vi "simulacao_robo_movel_old.vi"() -> ()   [LabVIEW 2013]
uses:
  <vilib>/ptbypt/NI_PtbyPt.lvlib
panel:
  out "Posição":dbl(knob) scale=0.0..10.0
  out "Vi 2":dbl(graph)
  in  "Vi":dbl(knob) scale=0.0..10.0
  in  "stop":bool
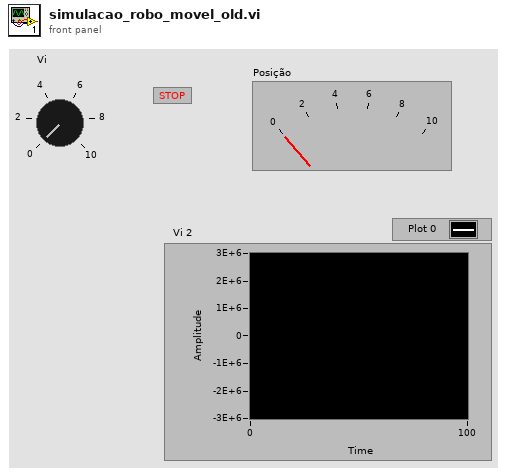
[diagram p1: front panel]
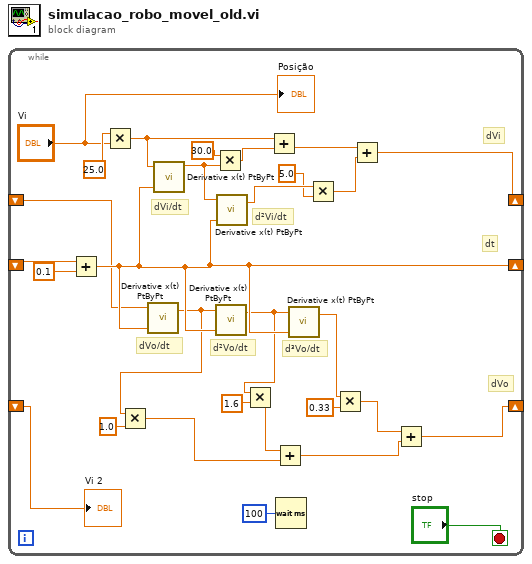
[diagram p0: block diagram]
diagram:
  n1 = while {
    shift-right: [w2] -> _
    shift-left: _ -> [w1]
    shift-right: [w15] -> _
    shift-left: _ -> [w17]
    shift-right: [w18] -> _
    shift-left: _ -> [w3]
    stop <- "stop" stop-if-true
    # "d³Vo/dt"
    # "dVo/dt"
    # "d²Vo/dt"
    # "dt"
    # "dVo"
    # "dVi/dt"
    # "d²Vi/dt"
    # "dVi"
    n2 = Add(x=w17, y=0.1 ("x")) -> (x+y=w15:dbl)
    n3 = Multiply(x=25.0 ("y"), y="Vi") -> (x*y=w26:dbl)
    n4 = call <vilib>:"Derivative x(t) PtByPt.vi"("dt"=w15, "V"=w3) -> ("dVi/dt"=w9:dbl)  [unwired: 2 in, 1 out]
    n5 = Multiply(x=w9, y=1.0) -> (x*y=w8:dbl)
    n6 = call <vilib>:"Derivative x(t) PtByPt.vi"("dt"=w15, "V"=w26) -> ("dVi/dt"=w23:dbl)  [unwired: 2 in, 1 out]
    n7 = Multiply(x=30.0, y=w23) -> (x*y=w25:dbl)
    n8 = call <vilib>:"Derivative x(t) PtByPt.vi"("dt"=w15, "V"=w9) -> ("dVi/dt"=w10:dbl)  [unwired: 2 in, 1 out]
    n9 = call <vilib>:"Derivative x(t) PtByPt.vi"("dt"=w15, "V"=w23) -> ("dVi/dt"=w22:dbl)  [unwired: 2 in, 1 out]
    n10 = Multiply(x=w10, y=1.6) -> (x*y=w7:dbl)
    n11 = Add(x=w26, y=w25) -> (x+y=w21:dbl)
    n12 = Add(x=w7, y=w8) -> (x+y=w5:dbl)
    n13 = Wait (ms)(milliseconds to wait=u32 100) -> ()  [unwired: 1 out]
    n14 = call <vilib>:"Derivative x(t) PtByPt.vi"("dt"=w15, "V"=w10) -> ("dVi/dt"=w11:dbl)  [unwired: 2 in, 1 out]
    n15 = Multiply(x=w22, y=5.0 ("x")) -> (x*y=w20:dbl)
    n16 = Multiply(x=w11, y=0.33) -> (x*y=w6:dbl)
    n17 = Add(x=w21, y=w20) -> (x+y=w18:dbl)
    n18 = Add(x=w6, y=w5) -> (x+y=w2:dbl)
    "Vi 2" <- w1
    "Posição" <- "Vi"
  }
